vi "Create Directory Structure.vi"(8 "error in (no error)":errorcluster, 9 "TargetRoot Name":string, 10 "Relative Directory Path":path, 11 "NIPKG Packager in":refnum<class "NIPKG Packager.lvclass">) -> (0 "error out":errorcluster, 2 "Target File Directory":path, 3 "NIPKG Packager out":refnum<class "NIPKG Packager.lvclass">, 4 "Data Directory":path)   [LabVIEW 2019, in "NIPKG Packager.lvclass"]
doc: "Creates the necessary directory structures within the build directory. The <b>Target File Directory</b> output is the location into which the files to be installed should be copied. A control file must be created at the <b>Control File Path</b>. The Data Directory is only needed if creating an instructions file."
uses:
  NIPKG Packager.lvclass
  NIPKG Packager.lvclass/NIPKG Packager.ctl
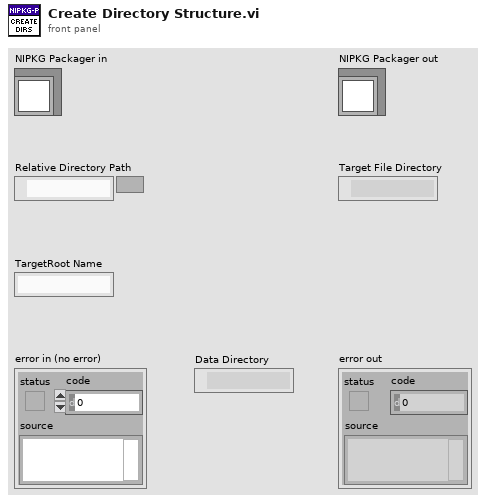
[diagram p1: front panel]
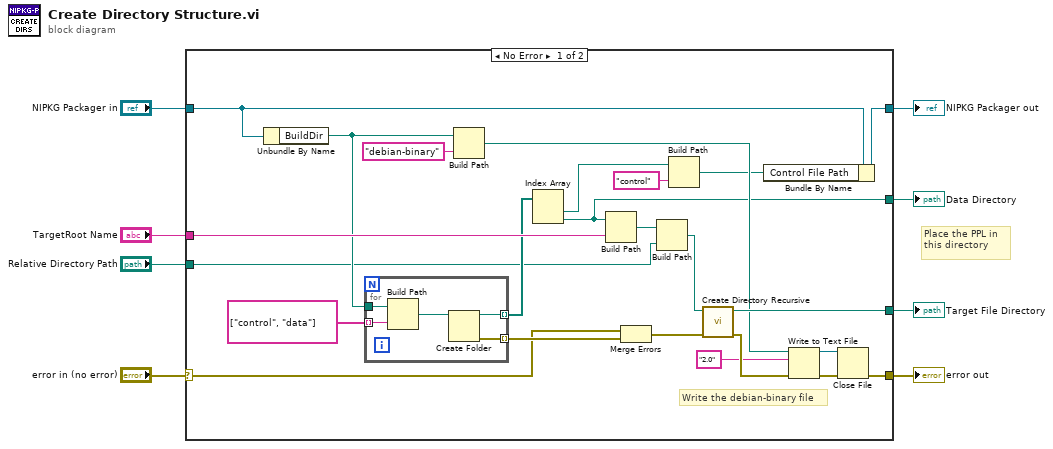
[diagram p0: block diagram]
diagram:
  # "Place the PPL in this directory"
  n1 = case shown="No Error" "error in (no error)" {
    selector: "error in (no error)" -> [w25 w39]
    tunnel: [w17 w39] -> w7
    tunnel: [w10 w38] -> w5
    tunnel: "NIPKG Packager in" -> [w32 w38]
    tunnel: "TargetRoot Name" -> [w30 _]
    tunnel: "Relative Directory Path" -> [w11 _]
    tunnel: [w24 _] -> w2
    tunnel: [w14 _] -> w1
    frame No Error {
      # "Write the debian-binary file"
      n2 = Unbundle By Name(w32) -> ("BuildDir"=w21:path)
      n3 = for {
        tunnel: w21 -> [w35]
        tunnel: string[] ["control", "data"] -> [w34] mode=indexing
        tunnel: [w33] -> w15 mode=indexing
        tunnel: [w37] -> w27 mode=indexing
        n4 = Build Path(base path=w35, name or relative path=w34) -> (appended path=w36:path)
        n5 = Create Folder(path (use dialog)=w36) -> (created path=w33:path, error out=w37:errorcluster)  [unwired: 2 in, 1 out]
      }
      n6 = Build Path(base path=w21, name or relative path="debian-binary") -> (appended path=w20:path)
      n7 = Index Array(array=w15) -> (element #1=w13:path, element #2=w14:path)  [unwired: 2 in]
      n8 = Build Path(base path=w14, name or relative path=w30) -> (appended path=w29:path)
      n9 = Merge Errors(w25, w27) -> (w26:errorcluster)
      n10 = Build Path(base path=w29, name or relative path=w11) -> (appended path=w28:path)
      n11 = Build Path(base path=w13, name or relative path="control") -> (appended path=w9:path)
      n12 = call <vilib>:"Create Directory Recursive.vi"("error in (no error)"=w26, "directory"=w28) -> ("error out"=w23:errorcluster, "directory copy"=w24:path)  [unwired: 3 in, 1 out]
      n13 = Bundle By Name(cluster=w32, "Control File Path"=w9) -> (w10:refnum<class "NIPKG Packager.lvclass">)
      n14 = Write to Text File(file (use dialog)=w20, text="2.0", error in=w23) -> (refnum out=w16:refnum<file>, error out=w22:errorcluster)  [unwired: 1 in, 1 out]
      n15 = Close File(refnum=w16, error in=w22) -> (error out=w17:errorcluster)  [unwired: 1 out]
    }
    frame Error {
    }
  }
  "error out" <- w7
  "NIPKG Packager out" <- w5
  "Target File Directory" <- w2
  "Data Directory" <- w1
